vi "AmmeterTest.vi"() -> ()   [LabVIEW 2012]
uses:
  Agilent 34401.lvlib
panel:
  out "read":u32
  out "trigger":u32
  out "total":u32
  out "Measurements":dbl[](array[numeric])
  in  "stop":bool
  out "error out":errorcluster
  in  "error in (no error)":errorcluster
  in  "VISA resource name":refnum<visa-resource-name>
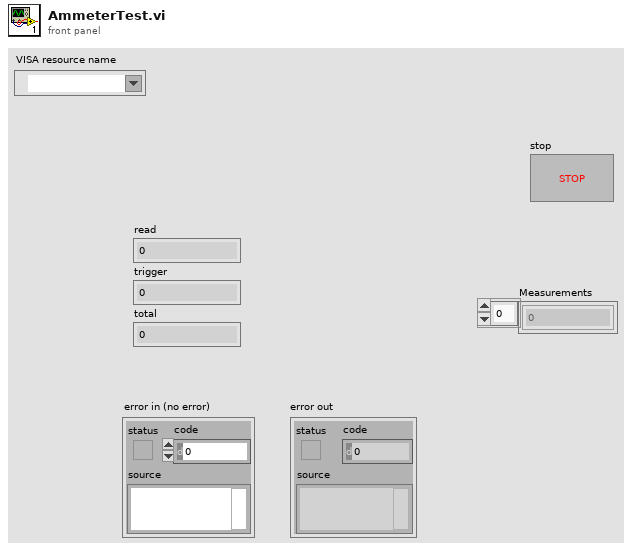
[diagram p1: front panel]
types:
  T1 = cluster{"Baud Rate":u32, "Parity":u16, "Data Bits":u16}
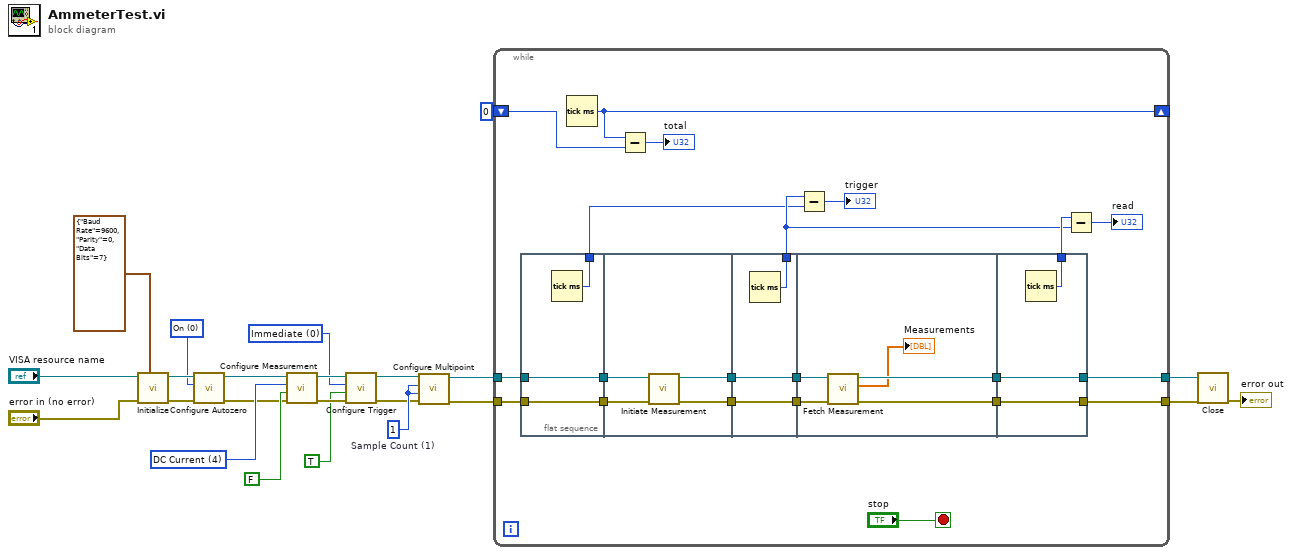
[diagram p0: block diagram]
diagram:
  w2 = u16 0 items=["On", "Off", "Once"] ("Autozero  (0: On)")
  w14 = 1  # Sample Count (1)
  w15 = u16 0 items=["Immediate", "Software (Bus)", "External", "Internal"] ("Trigger Source (0: Immediate)")
  w19 = u16 4 items=["DC Voltage", "AC Voltage", "2 - Wire Resistance", "4 - Wire Resistance", "DC Current", "AC Current", "Frequency", "Period", "Continuity", "Diode Checking", "VDC:VDC Ratio", "Temperature", "Capacitance"] ("Function (0: DC Voltage)")
  n1 = call "Initialize.vi"("Serial Configuration"=T1 {"Baud Rate"=9600, "Parity"=0, "Data Bits"=7}, "error in (no error)"="error in (no error)", "VISA resource name"="VISA resource name") -> ("error out"=w4:errorcluster, "VISA resource name out"=w6:refnum<visa-resource-name>)  [unwired: 7 in]
  n2 = call "Configure Autozero.vi"("error in (no error)"=w4, "Autozero  (0: On)"=w2, "VISA resource name"=w6) -> ("error out"=w3:errorcluster, "VISA resource name out"=w5:refnum<visa-resource-name>)  [unwired: 7 in]
  n3 = call "Configure Measurement.vi"("error in (no error)"=w3, "Enable Auto Range (T: Enable)"=FALSE, "Function (0: DC Voltage)"=w19, "VISA resource name"=w5) -> ("error out"=w16:errorcluster, "VISA resource name out"=w17:refnum<visa-resource-name>)  [unwired: 6 in]
  n4 = call "Configure Trigger.vi"("error in (no error)"=w16, "Enable Auto Delay (T: Enable)"=TRUE, "Trigger Source (0: Immediate)"=w15, "VISA resource name"=w17) -> ("error out"=w12:errorcluster, "VISA resource name out"=w13:refnum<visa-resource-name>)  [unwired: 6 in]
  n5 = call "Configure Multipoint.vi"("error in (no error)"=w12, "Sample Count (1)"=w14, "Trigger Count (1)"=w14, "VISA resource name"=w13) -> ("error out"=w8:errorcluster, "VISA resource name out"=w9:refnum<visa-resource-name>)  [unwired: 6 in]
  n6 = while {
    tunnel: [w43] -> w11
    tunnel: [w42] -> w10
    tunnel: w9 -> [w38]
    tunnel: w8 -> [w37]
    shift-right: [w39] -> _
    shift-left: u32 0 -> [w40]
    stop <- "stop" stop-if-true
    n7 = flat-sequence {
      tunnel: w37 -> [w46]
      tunnel: w38 -> [w47]
      tunnel: [w47] -> w30
      tunnel: [w46] -> w29
      tunnel: [w45] -> w26
      tunnel: [w50] -> w34
      tunnel: [w48] -> w32
      tunnel: w30 -> [w51]
      tunnel: w29 -> [w49]
      tunnel: w34 -> [w54]
      tunnel: [w54] -> w33
      tunnel: w32 -> [w53]
      tunnel: [w53] -> w31
      tunnel: [w52] -> w27
      tunnel: w33 -> [w56]
      tunnel: w31 -> [w55]
      tunnel: [w59] -> w36
      tunnel: [w58] -> w35
      tunnel: [w61] -> w42
      tunnel: [w62] -> w43
      tunnel: w36 -> [w62]
      tunnel: w35 -> [w61]
      tunnel: [w60] -> w28
      frame #0 {
        n8 = Tick Count (ms)() -> (millisecond timer value=w45:u32)
      }
      frame #1 {
        n9 = call "Initiate Measurement.vi"("error in (no error)"=w49, "VISA resource name"=w51) -> ("error out"=w48:errorcluster, "VISA resource name out"=w50:refnum<visa-resource-name>)  [unwired: 8 in]
      }
      frame #2 {
        n10 = Tick Count (ms)() -> (millisecond timer value=w52:u32)
      }
      frame #3 {
        n11 = call "Fetch Measurement.vi"("error in (no error)"=w55, "VISA resource name"=w56) -> ("error out"=w58:errorcluster, "Measurements"=→"Measurements":dbl[], "VISA resource name out"=w59:refnum<visa-resource-name>)  [unwired: 6 in, 1 out]
      }
      frame #4 {
        n12 = Tick Count (ms)() -> (millisecond timer value=w60:u32)
      }
    }
    n13 = Tick Count (ms)() -> (millisecond timer value=w39:u32)
    n14 = Subtract(x=w39, y=w40) -> (x-y=→"total":u32)
    n15 = Subtract(x=w27, y=w26) -> (x-y=→"trigger":u32)
    n16 = Subtract(x=w28, y=w27) -> (x-y=→"read":u32)
  }
  n17 = call "Close.vi"("error in (no error)"=w10, "VISA resource name"=w11) -> ("error out"=→"error out":errorcluster)  [unwired: 9 in]
